vi "receive data.vi"(0 "Serial port asssistant model in":refnum<class "Serial port assistant model.lvclass">, 11 "error in (no error)":errorcluster) -> (15 "error out":errorcluster)   [LabVIEW 2022 SP3, in "Serial port assistant model.lvlib" / "Serial port assistant model.lvclass"]
uses:
  Serial port assistant model.lvclass
  Serial port assistant model.lvclass/Serial port assistant model.ctl
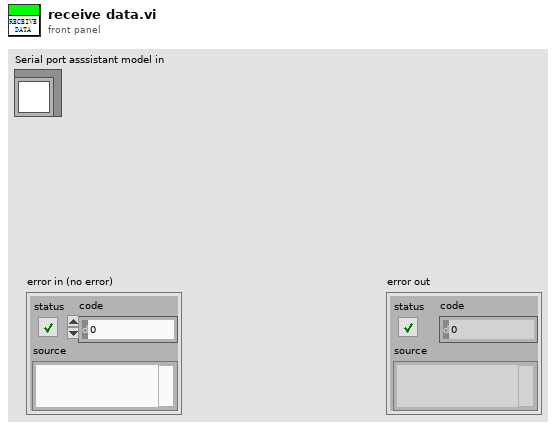
[diagram p1: front panel]
types:
  T1 = cluster{"changed data":string, "receive time":string, "data has been received":string}
  T2 = typedef "Rendezvous RefNum" = refnum<k1>
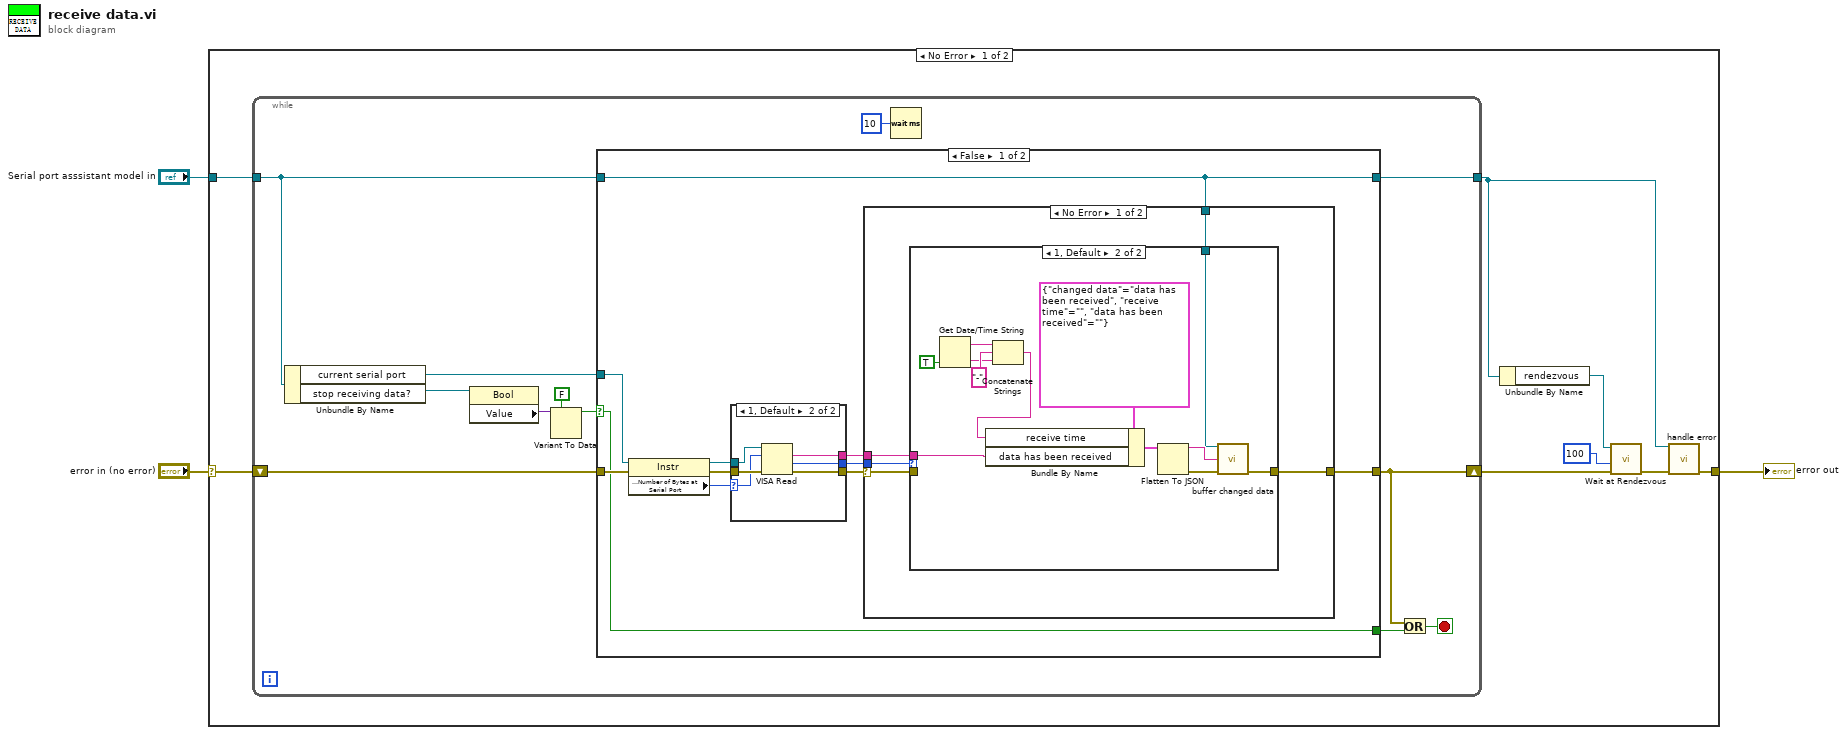
[diagram p0: block diagram]
diagram:
  n1 = case shown="No Error" "error in (no error)" {
    selector: "error in (no error)" -> [w10 w64]
    tunnel: "Serial port asssistant model in" -> [w11 _]
    tunnel: [w5 w64] -> w1
    frame No Error {
      n2 = while {
        tunnel: w11 -> [w18]
        shift-right: [w16] -> w7
        shift-left: w10 -> [w22]
        tunnel: [w12] -> w4
        stop <- w23 stop-if-true
        n3 = Unbundle By Name(w18) -> ("current serial port"=w14:refnum<visa-resource-name>, "stop receiving data?"=w19:refnum<vi>)
        n4 = property class="Bool"(reference=w19) -> ("Value"=w21:variant)  [unwired: 1 in, 2 out]
        n5 = Variant To Data(type=FALSE, Variant=w21) -> (data=w17:bool)  [unwired: 1 in, 1 out]
        n6 = case shown="False" w17 {
          selector: w17 -> [w26 w62]
          tunnel: w18 -> [w24 w61]
          tunnel: w22 -> [w28 w63]
          tunnel: [w27 w63] -> w16
          tunnel: [w26 w62] -> w15
          tunnel: w14 -> [w25 _]
          tunnel: [w24 w61] -> w12
          frame False {
            n7 = property class="Instr"(reference=w25, error in=w28) -> (reference out=w33:refnum<visa-resource-name>, error out=w34:errorcluster, "Serial Settings:Number of Bytes at Serial Port"=w31:u32)
            n8 = case shown="1, Default" w31 {
              selector: w31 -> [_ w38]
              tunnel: w34 -> [w35 w41]
              tunnel: w33 -> [_ w40]
              tunnel: [w35 w39] -> w32
              tunnel: [_ w37] -> w30
              tunnel: [_ w36] -> w29
              frame 0 {
              }
              frame 1, Default {
                n9 = VISA Read(VISA resource name=w40, byte count=w38, error in (no error)=w41) -> (read buffer=w37:string, return count=w36:u32, error out=w39:errorcluster)  [unwired: 1 out]
              }
            }
            n10 = case shown="No Error" w32 {
              selector: w32 -> [w42 w60]
              tunnel: w30 -> [w45 _]
              tunnel: w29 -> [w46 _]
              tunnel: [w44 w60] -> w27
              tunnel: w24 -> [w43 _]
              frame No Error {
                n11 = case shown="1, Default" w46 {
                  tunnel: w45 -> [_ w53]
                  tunnel: [w47 w57] -> w44
                  tunnel: w43 -> [_ w56]
                  tunnel: w42 -> [w47 _]
                  frame 0 {
                  }
                  frame 1, Default {
                    n12 = Get Date/Time String(want seconds? (F)=TRUE) -> (date string=w51:string, time string=w49:string)  [unwired: 2 in]
                    n13 = Concatenate Strings(w51, "-" ("string"), w49) -> (w48:string)
                    n14 = Bundle By Name(cluster=T1 {"changed data"="data has been received", "receive time"="", "data has been received"=""}, "receive time"=w48, "data has been received"=w53) -> (w54:T1)
                    n15 = Flatten To JSON(anything=w54) -> (JSON string=w58:string, 11:w59:errorcluster)  [unwired: 2 in]
                    n16 = call "buffer changed data.vi"("Serial port asssistant model in"=w56, "changed data"=w58, "error in (no error)"=w59) -> ("error out"=w57:errorcluster)  [unwired: 11 in, 1 out]
                  }
                }
              }
              frame Error {
              }
            }
          }
          frame True {
          }
        }
        n17 = Wait (ms)(milliseconds to wait=u32 10) -> ()  [unwired: 1 out]
        n18 = Or(x=w16, y=w15) -> (x .or. y?=w23:bool)
      }
      n19 = Unbundle By Name(w4) -> ("rendezvous"=w9:T2)
      n20 = call <vilib>:"Wait at Rendezvous.vi"("error in (no error)"=w7, "ms timeout (-1)"=100, "rendezvous"=w9) -> ("error out"=w6:errorcluster)  [unwired: 2 in, 2 out]
      n21 = call "handle error.vi"("Serial port assistant model in"=w4, "error in (no error)"=w6) -> ("error out"=w5:errorcluster)  [unwired: 12 in, 1 out]
    }
    frame Error {
    }
  }
  "error out" <- w1
